vi "View.vi"(11 "simple_html_chat_ui":refnum<class "simple_html_chat_ui.lvclass">) -> ()   [LabVIEW 2020, in "simple_html_chat_ui.lvclass"]
uses:
  simple_html_chat_ui.lvclass
  typedefs/queue_data.ctl
  simple_html_chat_ui.lvclass/simple_html_chat_ui.ctl
  D:/Personal/LabVIEW LLMs/src/user_interfaces/simple_html_chat_ui/assembly_support/Microsoft.Web.WebView2.Core.dll
  assembly_support/Microsoft.Web.WebView2.Core.dll
  typedefs/data_cluster.ctl
  <vilib>/MediaMongrels Ltd/WebSockets/WebSockets/WebSocket Server/WebSocket Server.lvclass
  models/message_text/message_text.lvclass
  D:/Personal/LabVIEW LLMs/src/models/abstract_message_base/abstract_message_base.lvclass
  models/message_text/create_text_message.vi
  <vilib>/addons/Tools/Unicode/UTF8 Tools.lvlib
  D:/Personal/LabVIEW LLMs/src/user_interfaces/simple_html_chat_ui/assembly_support/Microsoft.Web.WebView2.WinForms.dll
  assembly_support/Microsoft.Web.WebView2.WinForms.dll
panel:
  in  "WebView":refnum<k24>(container)
  out "error out":errorcluster
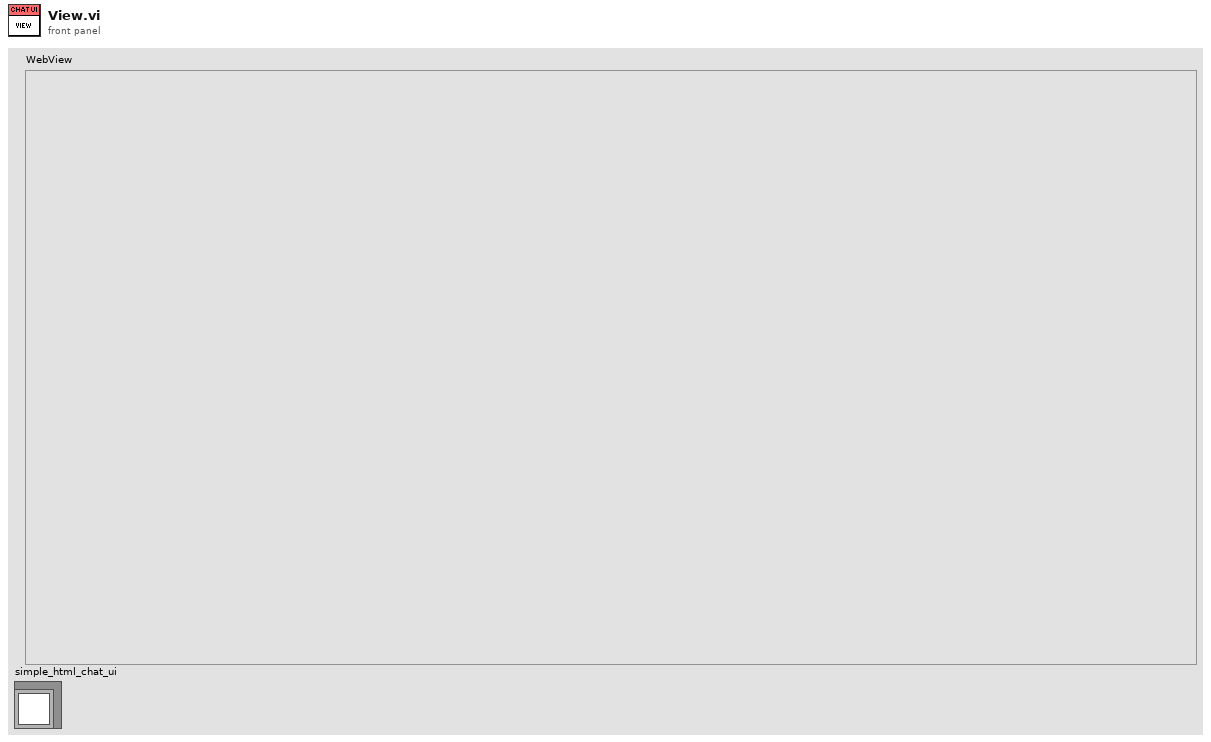
[diagram p1: front panel]
types:
  T1 = typedef "simple_html_chat_ui.lvclass/queue_data.ctl" = cluster{"State":string, "Data":variant}
  T2 = typedef "simple_html_chat_ui.lvclass/data_cluster.ctl" = cluster{"WS Connection":refnum<class "WebSocket Server.lvclass">}
  T3 = typedef "simple_html_chat_ui.lvclass/app_events.ctl" = cluster{"Exit":refnum<user-event>, "Publish data event":refnum<user-event>}
  T4 = typedef "simple_html_chat_ui.lvclass/web_events.ctl" = cluster{"User prompt":refnum<user-event>, "Clear history":refnum<user-event>}
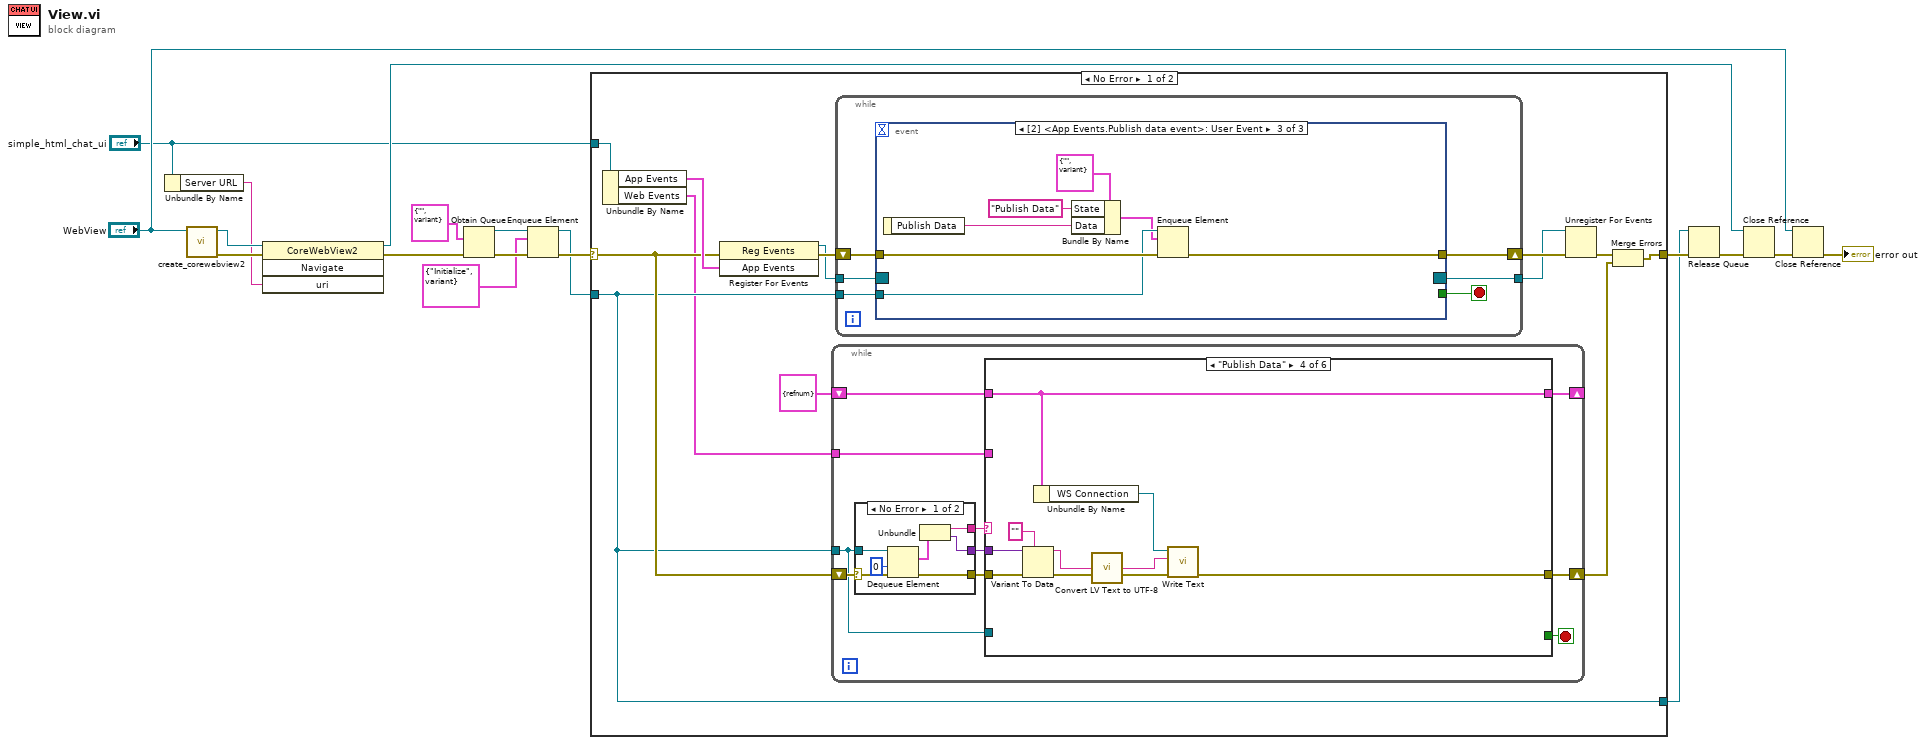
[diagram p0: block diagram]
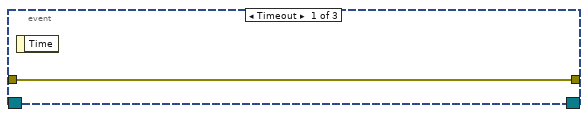
[diagram p2: hidden frame]
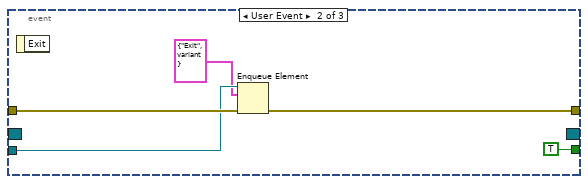
[diagram p3: hidden frame]
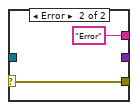
[diagram p4: hidden frame]
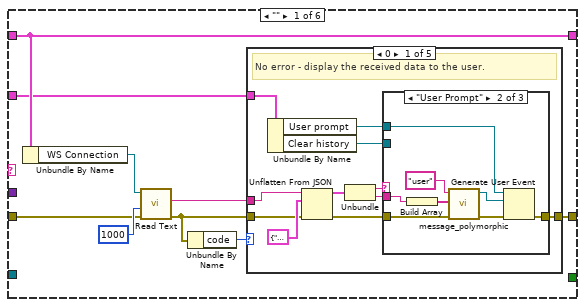
[diagram p5: hidden frame]
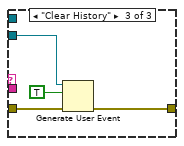
[diagram p7: hidden frame]
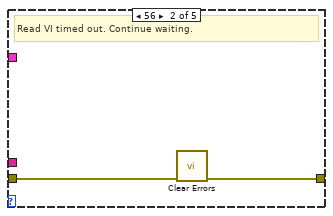
[diagram p8: hidden frame]
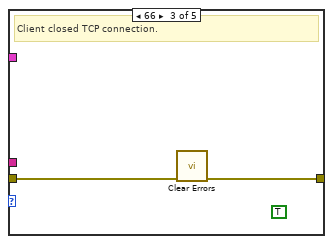
[diagram p9: hidden frame]
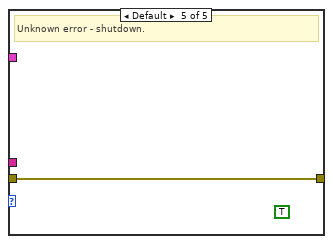
[diagram p11: hidden frame]
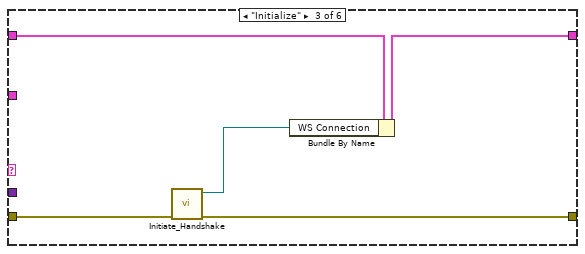
[diagram p13: hidden frame]
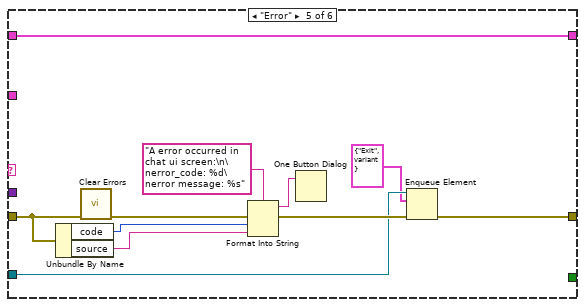
[diagram p14: hidden frame]
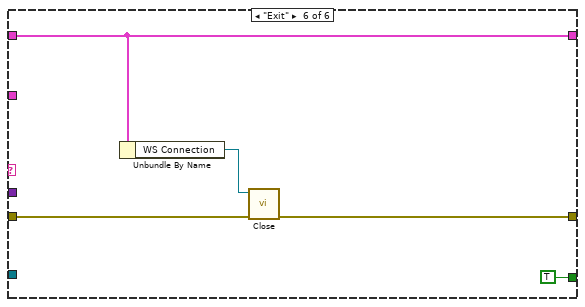
[diagram p15: hidden frame]
diagram:
  n1 = Unbundle By Name("simple_html_chat_ui") -> ("Server URL"=w6:string)
  n2 = call "create_corewebview2.vi"("WebView2"="WebView") -> ("error out"=w8:errorcluster, "CoreWebView2"=w7:refnum<k24>)  [unwired: 9 in]
  n3 = invoke class="CoreWebView2" method="Navigate"(reference=w7, error in=w8, "uri"=w6) -> (reference out=w14:refnum<k24>, error out=w5:errorcluster)  [unwired: 1 in, 2 out]
  n4 = Obtain Queue(element data type=T1 {"State"="", "Data"=variant} ("Cluster"), error in (no error)=w5) -> (queue out=w2:refnum<queue>, error out=w3:errorcluster)  [unwired: 3 in, 1 out]
  n5 = Enqueue Element(queue=w2, element=T1 {"State"="Initialize", "Data"=variant} ("Cluster"), error in (no error)=w3) -> (queue out=w12:refnum<queue>, error out=w15:errorcluster)  [unwired: 1 in, 1 out]
  n6 = case shown="No Error" w15 {
    selector: w15 -> [w24 w143]
    tunnel: [w22 w143] -> w11
    tunnel: "simple_html_chat_ui" -> [w28 _]
    tunnel: w12 -> [w20 w142]
    tunnel: [w20 w142] -> w9
    frame No Error {
      n7 = Unbundle By Name(w28) -> ("App Events"=w26:T3, "Web Events"=w19:T4)
      n8 = register-events(error in=w24, w26) -> (reference out=w25:refnum<event-registration>, error out=w27:errorcluster)  [unwired: 1 in]
      n9 = while {
        tunnel: w20 -> [w53]
        shift-right: [w56] -> w21
        shift-left: w24 -> [w60]
        shift-right: [w54] -> _
        shift-left: T2 {"WS Connection"=refnum} ("Data Cluster") -> [w55]
        tunnel: w19 -> [w51]
        stop <- w52 stop-if-true
        n10 = case shown="No Error" w60 {
          selector: w60 -> [w67 w69]
          tunnel: w53 -> [w66 _]
          tunnel: [w64 w69] -> w59
          tunnel: [w63 "Error" ("State")] -> w58
          tunnel: [w62 _] -> w57
          frame No Error {
            n11 = Dequeue Element(queue=w66, timeout in ms (-1)=0, error in (no error)=w67) -> (element=w65:T1, error out=w64:errorcluster)  [unwired: 2 out]
            n12 = Unbundle(w65) -> ("State"=w63:string, "Data"=w62:variant)
          }
          frame Error {
          }
        }
        n13 = case shown="\"Publish Data\"" w58 {
          tunnel: w59 -> [w76 w109 w115 w125 w135 w139]
          tunnel: w57 -> [_ _ _ w124 _ _]
          tunnel: [w72 w109 w114 w121 w128 w138] -> w56
          tunnel: w55 -> [w78 w110 w113 w120 w136 w140]
          tunnel: [w78 w110 w111 w120 w136 w140] -> w54
          tunnel: w53 -> [_ _ _ _ w127 _]
          tunnel: [_ _ _ _ _ TRUE] -> w52
          tunnel: w51 -> [w70 _ _ _ _ _]
          frame "" {
            n14 = Unbundle By Name(w78) -> ("WS Connection"=w75:refnum<class "WebSocket Server.lvclass">)
            n15 = call-dynamic "Read Text.vi"("error in (no error)"=w76, "timeout ms (5000)"=1000 ("timeout ms (25000)"), "WebSocket in"=w75) -> ("error out"=w74:errorcluster, "Data"=w71:string)  [unwired: 6 in, 1 out]
            n16 = Unbundle By Name(w74) -> ("code"=w73:i32)
            n17 = case shown="0" w73 {
              tunnel: w74 -> [w87 w104 w106 w107 w108]
              tunnel: [w80 w103 w105 w107 w108] -> w72
              tunnel: w71 -> [w86 _ _ _ _]
              tunnel: w70 -> [w82 _ _ _ _]
              frame 0 {
                # "No error - display the received data to the user."
                n18 = Unbundle By Name(w82) -> ("User prompt"=w81:refnum<user-event>, "Clear history"=w79:refnum<user-event>)
                n19 = Unflatten From JSON(JSON string=w86, type and defaults=cluster{"key":string, "data":string} {"key"="", "data"=""}, error in (no error)=w87) -> (value=w88:cluster{"key":string, "data":string}, error out=w85:errorcluster)  [unwired: 4 in]
                n20 = Unbundle(w88) -> ("key"=w84:string, "data"=w83:string)
                n21 = case shown="\"User Prompt\"" w84 {
                  tunnel: w85 -> [w90 w93 w102]
                  tunnel: w83 -> [_ w92 _]
                  tunnel: w81 -> [_ w98 _]
                  tunnel: [w90 w97 w101] -> w80
                  tunnel: w79 -> [_ _ w100]
                  frame Default {
                    # "#todo - generate error for undefined events"
                  }
                  frame "User Prompt" {
                    n22 = Build Array(w92) -> (w95:string[])
                    n23 = call-poly "message_polymorphic.vi"("error in (no error)"=w93, "content"=w95, "role"="user") -> ("error out"=w94:errorcluster, "message_text out"=w91:refnum<class "message_text.lvclass">)  [unwired: 7 in]
                    n24 = Generate User Event(user event=w98, event data cluster=w91, error in=w94) -> (error out=w97:errorcluster)  [unwired: 1 in, 1 out]
                  }
                  frame "Clear History" {
                    n25 = Generate User Event(user event=w100, event data cluster=TRUE ("event data"), error in=w102) -> (error out=w101:errorcluster)  [unwired: 1 in, 1 out]
                  }
                }
              }
              frame 56 {
                # "Read VI timed out. Continue waiting."
                n26 = call <vilib>:"Clear Errors.vi"("error in (no error)"=w104) -> ("error out"=w103:errorcluster)  [unwired: 5 in, 1 out]
              }
              frame 66 {
                (unwired) TRUE
                # "Client closed TCP connection."
                n27 = call <vilib>:"Clear Errors.vi"("error in (no error)"=w106) -> ("error out"=w105:errorcluster)  [unwired: 5 in, 1 out]
              }
              frame 6066 {
                # "Error 6066: Client requested to close the connection. Send 'close' opcode."
              }
              frame Default {
                (unwired) TRUE
                # "Unknown error - shutdown."
              }
            }
          }
          frame Default {
          }
          frame "Initialize" {
            n28 = call "Initiate_Handshake.vi"("error in"=w115) -> ("error out"=w114:errorcluster, "WebSocket Connection out"=w112:refnum<class "WebSocket Server.lvclass">)  [unwired: 8 in]
            n29 = Bundle By Name(cluster=w113, "WS Connection"=w112) -> (w111:T2)
          }
          frame "Publish Data" {
            n30 = Variant To Data(error in=w125, type="", Variant=w124) -> (data=w117:string, error out=w122:errorcluster)
            n31 = Unbundle By Name(w120) -> ("WS Connection"=w119:refnum<class "WebSocket Server.lvclass">)
            n32 = call <vilib>:"Convert LV Text to UTF-8.vi"("LV Text"=w117, "error in"=w122) -> ("UTF-8 Text"=w116:string, "error out"=w118:errorcluster)  [unwired: 12 in]
            n33 = call-dynamic "Write Text.vi"("error in (no error)"=w118, "String Data"=w116, "WebSocket in"=w119) -> ("error out"=w121:errorcluster)  [unwired: 7 in, 1 out]
          }
          frame "Error" {
            n34 = Unbundle By Name(w135) -> ("code"=w132:i32, "source"=w131:string)
            n35 = call <vilib>:"Clear Errors.vi"("error in (no error)"=w135) -> ("error out"=w134:errorcluster)  [unwired: 5 in, 1 out]
            n36 = Format Into String(format string="A error occurred in chat ui screen:\n\nerror_code: %d\nerror message: %s", error in=w134, w132, w131) -> (resulting string=w130:string, error out=w129:errorcluster)  [unwired: 1 in]
            n37 = One Button Dialog(message=w130) -> ()  [unwired: 1 in, 1 out]
            n38 = Enqueue Element(queue=w127, element=T1 {"State"="Exit", "Data"=variant} ("Cluster"), error in (no error)=w129) -> (error out=w128:errorcluster)  [unwired: 1 in, 2 out]
          }
          frame "Exit" {
            n39 = Unbundle By Name(w140) -> ("WS Connection"=w137:refnum<class "WebSocket Server.lvclass">)
            n40 = call-dynamic "Close.vi"("error in (no error)"=w139, "WebSocket in"=w137) -> ("error out"=w138:errorcluster)  [unwired: 9 in]
          }
        }
      }
      n41 = while {
        shift-right: [w36] -> w31
        shift-left: w27 -> [w37]
        tunnel: [w35] -> w30
        tunnel: w25 -> [w34]
        tunnel: w20 -> [w33]
        stop <- w32 stop-if-true
        n42 = event shown="[2] <App Events.Publish data event>: User Event" {
          selector: w34 -> [_ _ _]
          dyn-events: [_ _ _] -> w35
          timeout: _ -> [_ _ _]
          tunnel: w37 -> [w38 w43 w49]
          tunnel: [w38 w42 w50] -> w36
          tunnel: w33 -> [_ w41 w48]
          tunnel: [_ TRUE _] -> w32
          event Timeout {
            n43 = event-data() -> ()  [unwired: 1 in, 1 out]
          }
          event User Event {
            n44 = event-data() -> ()  [unwired: 1 in, 1 out]
            n45 = Enqueue Element(queue=w41, element=T1 {"State"="Exit", "Data"=variant} ("Cluster"), error in (no error)=w43) -> (error out=w42:errorcluster)  [unwired: 1 in, 2 out]
          }
          event User Event {
            n46 = event-data() -> ("Publish Data"=w45:string)  [unwired: 1 in]
            n47 = Bundle By Name(cluster=T1 {"State"="", "Data"=variant} ("Cluster"), "State"="Publish Data", "Data"=w45) -> (w44:T1)
            n48 = Enqueue Element(queue=w48, element=w44, error in (no error)=w49) -> (error out=w50:errorcluster)  [unwired: 1 in, 2 out]
          }
        }
      }
      n49 = Unregister For Events(event registration refnum=w30, error in=w31) -> (error out=w29:errorcluster)
      n50 = Merge Errors(w29, w21) -> (w22:errorcluster)
    }
    frame Error {
    }
  }
  n51 = Release Queue(queue=w9, error in (no error)=w11) -> (error out=w10:errorcluster)  [unwired: 1 in, 2 out]
  n52 = Close Reference(reference=w14, error in (no error)=w10) -> (error out=w17:errorcluster)
  n53 = Close Reference(reference="WebView", error in (no error)=w17) -> (error out=→"error out":errorcluster)
